vi "BASE_Paths.vi"() -> ()   [LabVIEW 2017]
panel:
  out "path":path
  out "stripped path":path
  out "Application(my.exe) Directory Path":path
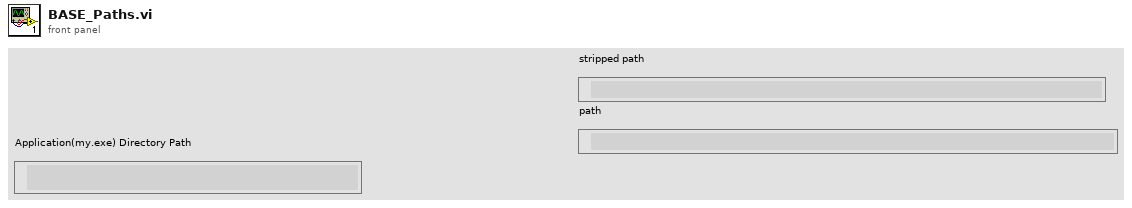
[diagram p1: front panel]
types:
  T1 = enum32{"invalid app kind", "Development System", "Run Time System", "Student Edition", "Embedded LabVIEW", "Evaluation", "Custom"}
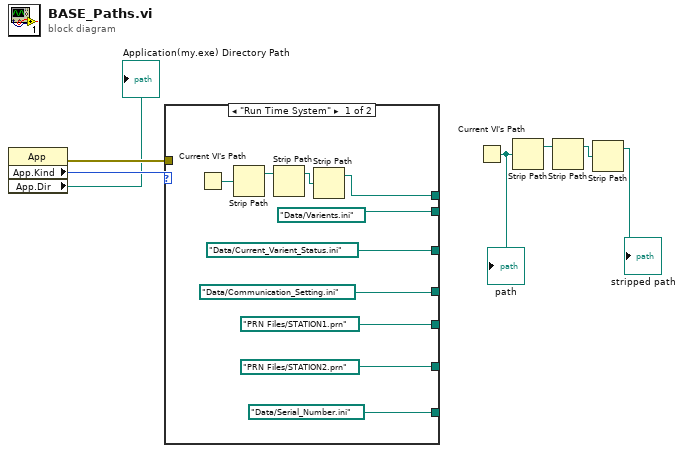
[diagram p0: block diagram]
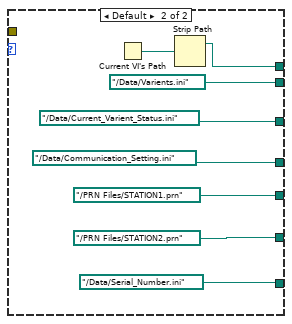
[diagram p2: hidden frame]
diagram:
  n1 = property class="App"() -> (error out=w6:errorcluster, "App.Kind"=w7:T1, "App.Dir"=→"Application(my.exe) Directory Path":path)  [unwired: 2 in, 1 out]
  n2 = case shown="\"Run Time System\"" w7 {
    tunnel: [path "Data/Varients.ini" ("path") path "../Data/Varients.ini" ("path")] -> _
    tunnel: [w13 w23] -> _
    tunnel: [path "Data/Current_Varient_Status.ini" ("path") path "../Data/Current_Varient_Status.ini" ("path")] -> _
    tunnel: [path "Data/Communication_Setting.ini" ("path") path "../Data/Communication_Setting.ini" ("path")] -> _
    tunnel: [path "PRN Files/STATION2.prn" ("path") path "../PRN Files/STATION2.prn" ("path")] -> _
    tunnel: w6 -> [_ _]
    tunnel: [path "PRN Files/STATION1.prn" ("path") path "../PRN Files/STATION1.prn" ("path")] -> _
    tunnel: [path "Data/Serial_Number.ini" ("path") path "../Data/Serial_Number.ini" ("path")] -> _
    frame "Run Time System" {
      n3 = Current VI's Path() -> (path=w16:path)
      n4 = Strip Path(path=w16) -> (stripped path=w15:path)  [unwired: 1 out]
      n5 = Strip Path(path=w15) -> (stripped path=w14:path)  [unwired: 1 out]
      n6 = Strip Path(path=w14) -> (stripped path=w13:path)  [unwired: 1 out]
    }
    frame Default {
      n7 = Current VI's Path() -> (path=w24:path)
      n8 = Strip Path(path=w24) -> (stripped path=w23:path)  [unwired: 1 out]
    }
  }
  n9 = Current VI's Path() -> (path=w4:path)
  "path" <- w4
  n10 = Strip Path(path=w4) -> (stripped path=w3:path)  [unwired: 1 out]
  n11 = Strip Path(path=w3) -> (stripped path=w2:path)  [unwired: 1 out]
  n12 = Strip Path(path=w2) -> (stripped path=→"stripped path":path)  [unwired: 1 out]
